vi "Configure Frequency Center Span.vi"(7 "Frequency Span (1E+6 Hz)":dbl=1000000.0, 8 "error in (no error)":errorcluster, 9 "Center Frequency (1E+6 Hz)":dbl=1000000.0, 10 "Channel (1)":i32=1, 11 "VISA resource name":refnum<visa-resource-name>) -> (0 "error out":errorcluster, 3 "VISA resource name out":refnum<visa-resource-name>)   [LabVIEW 2018, in "Keysight PNA Series.lvlib"]
doc: "Sets the center frequency and the frequency span of the analyzer."
uses:
  Keysight PNA Series.lvlib
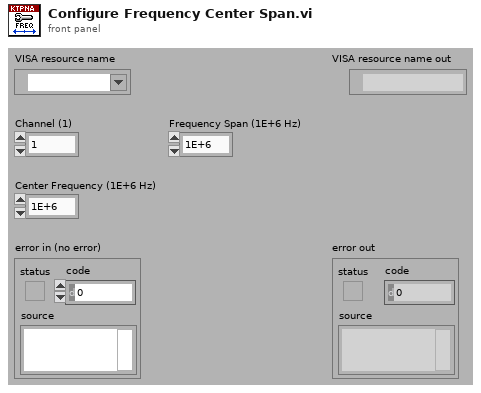
[diagram p1: front panel]
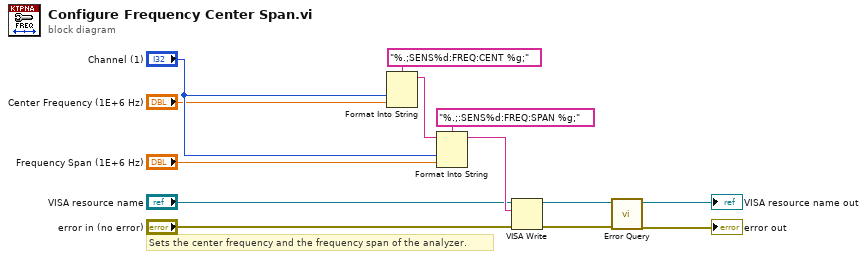
[diagram p0: block diagram]
diagram:
  # "Sets the center frequency and the frequency span of the analyzer."
  n1 = Format Into String(format string="%.;SENS%d:FREQ:CENT %g;", "Channel (1)", "Center Frequency (1E+6 Hz)") -> (resulting string=w10:string)  [unwired: 2 in, 1 out]
  n2 = Format Into String(format string="%.;:SENS%d:FREQ:SPAN %g;", initial string=w10, "Channel (1)", "Frequency Span (1E+6 Hz)") -> (resulting string=w7:string)  [unwired: 1 in, 1 out]
  n3 = VISA Write(VISA resource name="VISA resource name", write buffer=w7, error in (no error)="error in (no error)") -> (VISA resource name out=w4:refnum<visa-resource-name>, error out=w3:errorcluster)  [unwired: 1 out]
  n4 = call "Error Query.vi"("error in (no error)"=w3, "VISA resource name"=w4) -> ("error out"=→"error out":errorcluster, "VISA resource name out"=→"VISA resource name out":refnum<visa-resource-name>)  [unwired: 6 in, 2 out]
